vi "macro_TrajectoryConstraint_EllipRegion.vi"   [LabVIEW 2019, in "Trajectory_Library.lvlib"]
uses:
  Trajectory_Library.lvlib
types:
  T1 = typedef "Trajectory_Library.lvlib/ROTATION2D.ctl" = cluster{"VALUE":dbl, "COS":dbl, "SIN":dbl}
  T2 = typedef "WPILib_Math.lvlib/TRANSLATION2D.ctl" = cluster{"X":dbl, "Y":dbl}
  T3 = typedef "Trajectory_Library.lvlib/TRAJ_CONSTRAINT_MAX_VELOCITY.ctl" = cluster{"Max Velocity":dbl, "IM UNIQUE":bool}
  T4 = typedef "WPILib_Math.lvlib/TRAJ_CONSTRAINT_ELLIP_REGION.ctl" = cluster{"Center":T2, "Radii":T2, "Constraint":variant, "Constraint Type":T5, "IM UNIQUE":bool}
  T5 = typedef "WPILib_Math.lvlib/TRAJ_CONSTRAINT_TYPES_ENUM.ctl" = enum16{"UNDEFINED", "DIFF DRIVE KINEMATICS", "DIFF DRIVE VOLTAGE", "CENTRIPITAL ACCEL", "MECA DRIVE KINEMATICS", "SWERVE DRIVE KINEMATICS", "MAXIMUM VELOCITY", "ELLIPTICAL REGION", "RECTANGULAR REGION"}
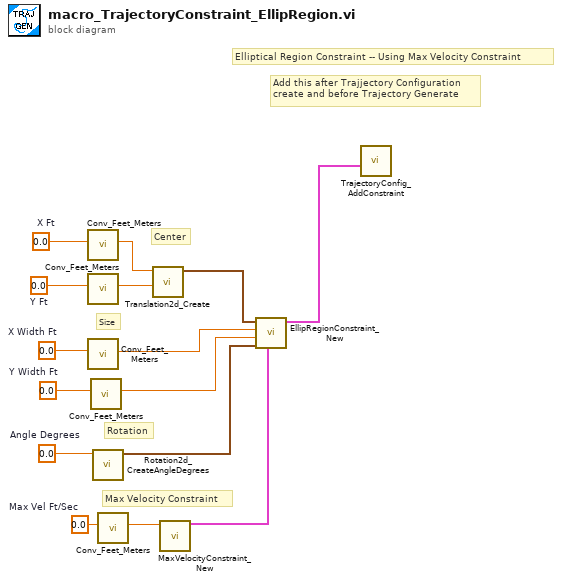
[diagram p0: block diagram]
diagram:
  w2 = 0.0  # Angle Degrees
  w8 = 0.0  # Max Vel Ft/Sec
  w11 = 0.0  # X Width Ft
  w10 = 0.0  # Y Width Ft
  w13 = 0.0  # X Ft
  w12 = 0.0  # Y Ft
  # "Rotation"
  # "Size"
  # "Max Velocity Constraint"
  # "Center"
  # "Elliptical Region Constraint -- Using Max Velocity Constraint"
  # "Add this after Trajjectory Configuration\ncreate and before Trajectory Generate"
  n1 = call "Conv_Feet_Meters.vi"("Feet"=w13) -> ("Meters"=w15:dbl)  [unwired: 10 in]
  n2 = call "Conv_Feet_Meters.vi"("Feet"=w12) -> ("Meters"=w14:dbl)  [unwired: 10 in]
  n3 = call "Conv_Feet_Meters.vi"("Feet"=w11) -> ("Meters"=w4:dbl)  [unwired: 10 in]
  n4 = call "Conv_Feet_Meters.vi"("Feet"=w10) -> ("Meters"=w3:dbl)  [unwired: 10 in]
  n5 = call "Rotation2d_CreateAngleDegrees.vi"("Angle_Degrees"=w2) -> ("ROTATION"=w1:T1)  [unwired: 10 in]
  n6 = call "Conv_Feet_Meters.vi"("Feet"=w8) -> ("Meters"=w9:dbl)  [unwired: 10 in]
  n7 = call "Translation2d_Create.vi"("Y"=w14, "X"=w15) -> ("TRANSLATION"=w5:T2)  [unwired: 9 in]
  n8 = call "MaxVelocityConstraint_New.vi"("Maximum Velocity"=w9) -> ("MAX_VELOCITY_CONSTRAINT"=w6:T3)  [unwired: 10 in]
  n9 = call "EllipRegionConstraint_New.vi"("Constraint Data Cluster"=w6, "Rotation"=w1, "Y Width"=w3, "X Width"=w4, "Center"=w5) -> ("ELLIP_REGION_CONSTRAINT"=w7:T4)  [unwired: 6 in]
  n10 = call "TrajectoryConfig_AddConstraint.vi"("Constraint"=w7) -> ()  [unwired: 10 in, 1 out]
